vi "Start Computation.vi"(8 "error in (no error)":errorcluster, 11 "VISA resource name":refnum<visa-resource-name>) -> (0 "error out":errorcluster, 3 "VISA resource name out":refnum<visa-resource-name>)   [LabVIEW 2020, in "Yokogawa GX Series.lvlib"]
doc: "Clears the computation data dropout display."
uses:
  <instrlib>/Yokogawa GX Series/Yokogawa GX Series.lvlib
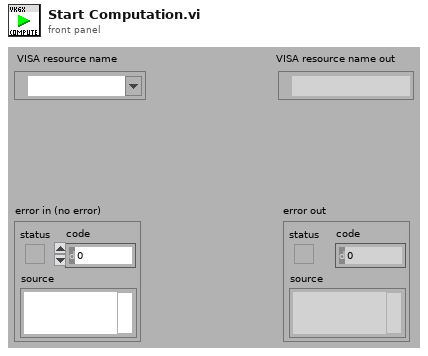
[diagram p1: front panel]
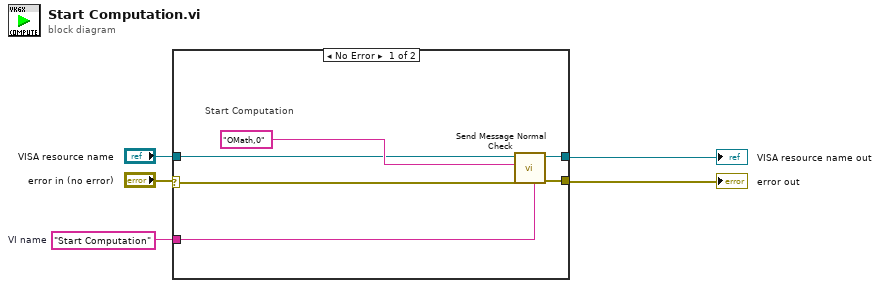
[diagram p0: block diagram]
diagram:
  w2 = "Start Computation"  # VI name
  n1 = case shown="No Error" "error in (no error)" {
    selector: "error in (no error)" -> [w6 w12]
    tunnel: "VISA resource name" -> [w7 w13]
    tunnel: [w11 w13] -> w4
    tunnel: [w10 w12] -> w3
    tunnel: w2 -> [w9 _]
    frame No Error {
      # "Start Computation"
      n2 = call <instrlib>:"Send Message Normal Check.vi"("Source (\"\")"=w9, "error in (no error)"=w6, "Send Message (\"\")"="OMath,0", "VISA resource name"=w7) -> ("error out"=w10:errorcluster, "VISA resource name out"=w11:refnum<visa-resource-name>)  [unwired: 2 in, 4 out]
    }
    frame Error {
    }
  }
  "error out" <- w3
  "VISA resource name out" <- w4
